vi "remote_fpga.vi"() -> ()   [LabVIEW 2018]
uses:
  packet_t.ctl
  packet_type_t.ctl
  spi_instructions.ctl
  seven_seg_digit.ctl
  grabber_register_addr.ctl
panel:
  out "unsigned byte array":u8[](array[numeric]) format="%x"
  out "Numeric":u8 format="%x"
  out "stop 3":bool
  in  "address":string="172.16.1.2"
  out "stop 2":bool
  in  "Colors [4]":cluster{u32, u32}[](array[cluster]) {"?" format="%x"}
  in  "stop":bool
  in  "Remote FPGA":enum32{"GPIO", "Page 2"}(tab)
  in  "Buttons":T1
  in  "SW7-0":bool[](array[boolean])=[FALSE, FALSE, FALSE, FALSE, FALSE, FALSE, FALSE, FALSE]
  in  "SW15-8":bool[](array[boolean])=[FALSE, FALSE, FALSE, FALSE, FALSE, FALSE, FALSE, FALSE]
  in  "Enable all":bool
  in  "Reset all":bool
  out "LED7-0":bool[](array[boolean])
  out "LED15-8":bool[](array[boolean])
  out "Digit":T2
  out "Digit 1":T2
  out "Digit 2":T2
  out "Digit 3":T2
  out "Digit 4":T2
  out "Digit 5":T2
  out "Digit 6":T2
  out "Digit 7":T2
  out "element":T3 {"instruction" items=["default"=0, "write"=173, "read"=237, "clear"=205]; "data" format="%x"; "address" format="%x"}
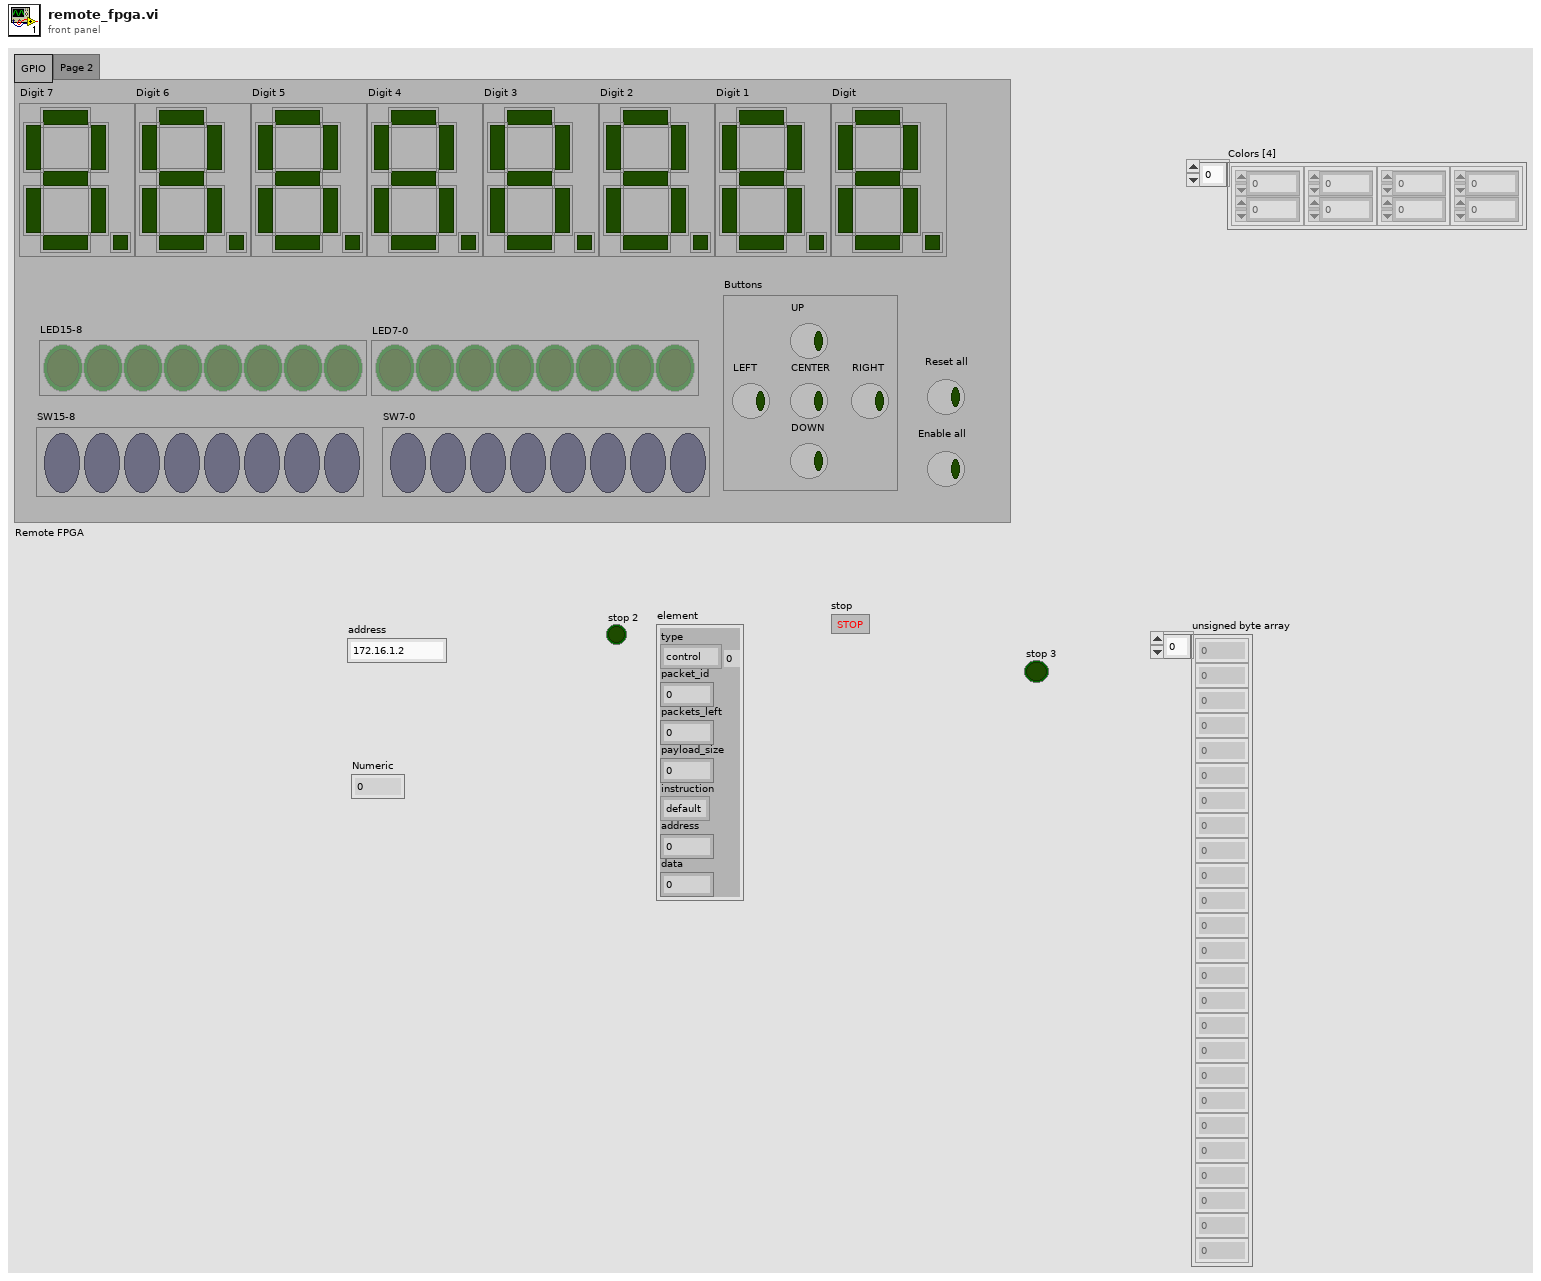
[diagram p1: front panel]
types:
  T1 = cluster{"CENTER":bool, "UP":bool, "LEFT":bool, "RIGHT":bool, "DOWN":bool}
  T2 = typedef "seven_seg_digit.ctl" = cluster{"DP":bool, "A":bool, "B":bool, "C":bool, "D":bool, "E":bool, "F":bool, "G":bool}
  T3 = typedef "packet_t.ctl" = cluster{"type":T4, "packet_id":u16, "packets_left":u16, "payload_size":u16, "instruction":T5, "address":u8, "data":u8}
  T4 = typedef "packet_type_t.ctl" = enum8{"control", "spi", "audio", "hdmi"}
  T5 = typedef "spi_instructions.ctl" = u8
  T6 = typedef "grabber_register_addr.ctl" = enum8{"rgb_data", "led_data_low", "led_data_high", "digit_0_data", "digit_1_data", "digit_2_data", "digit_3_data", "digit_4_data", "digit_5_data", "digit_6_data", "digit_7_data"}
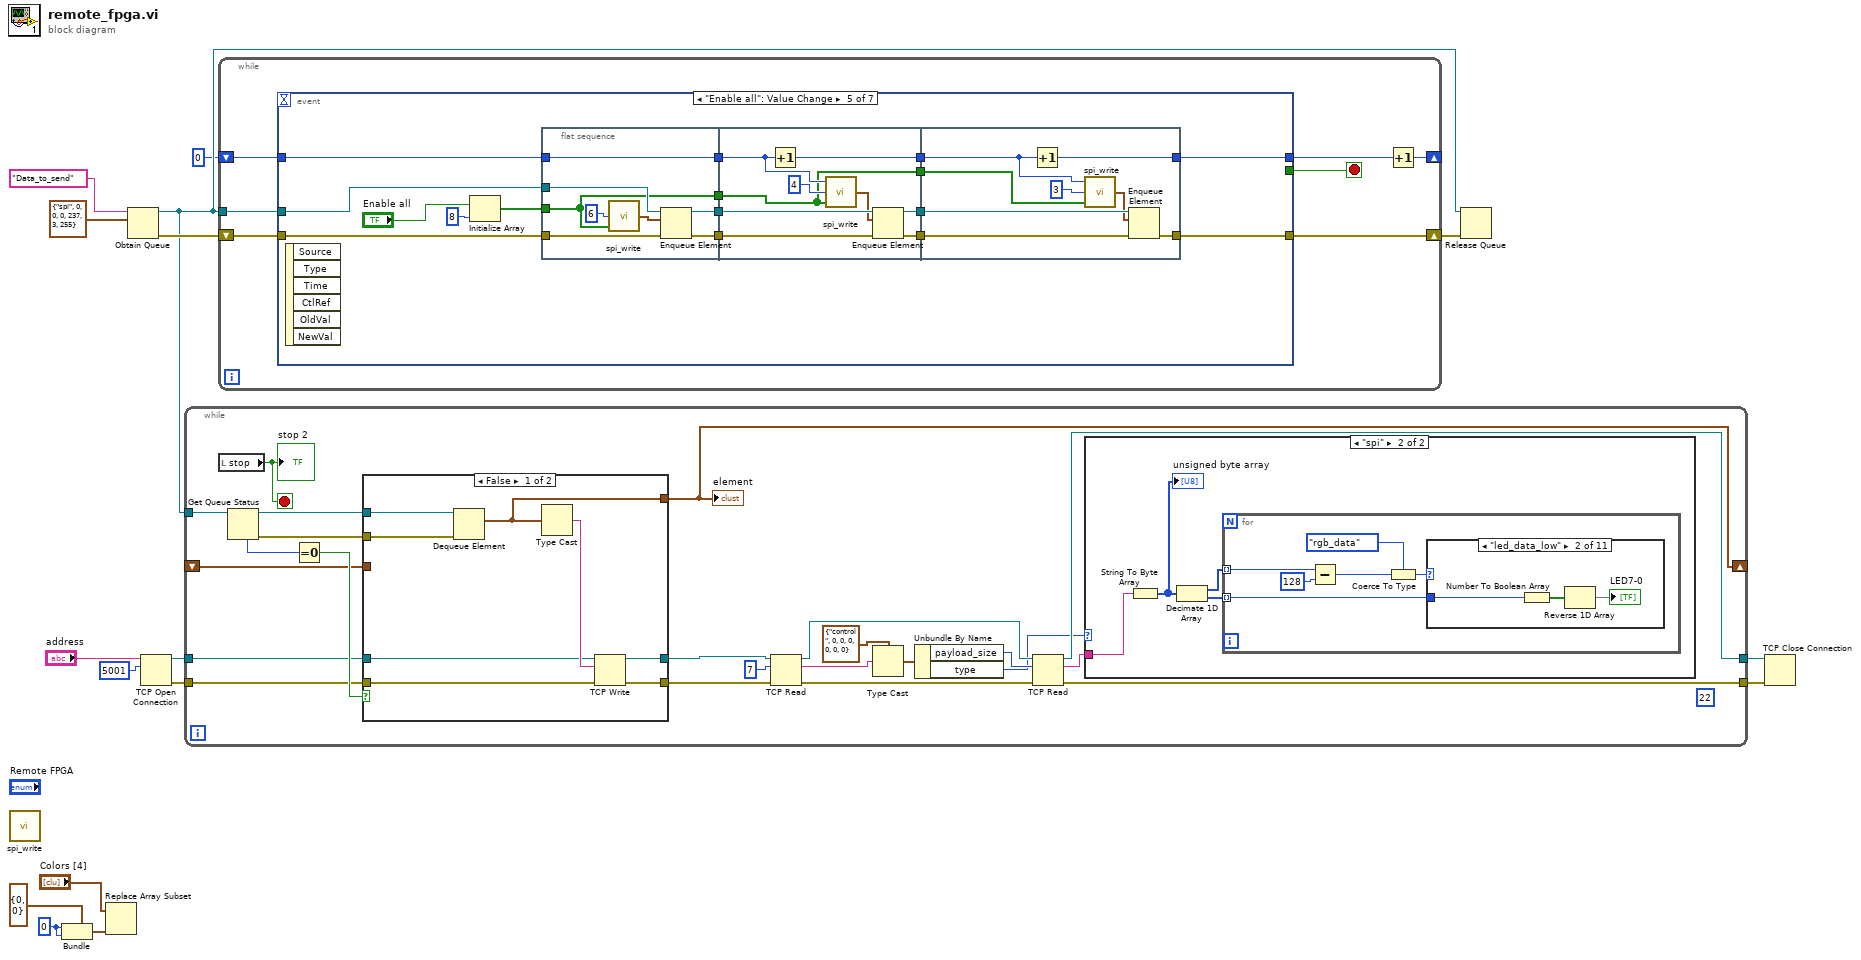
[diagram p0: block diagram]
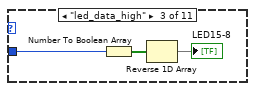
[diagram p4: hidden frame]
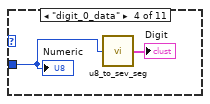
[diagram p5: hidden frame]
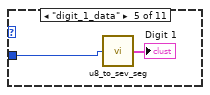
[diagram p6: hidden frame]
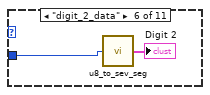
[diagram p7: hidden frame]
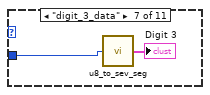
[diagram p8: hidden frame]
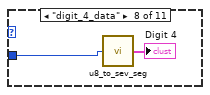
[diagram p9: hidden frame]
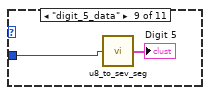
[diagram p10: hidden frame]
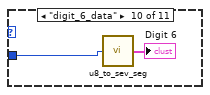
[diagram p11: hidden frame]
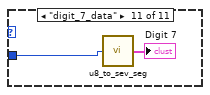
[diagram p12: hidden frame]
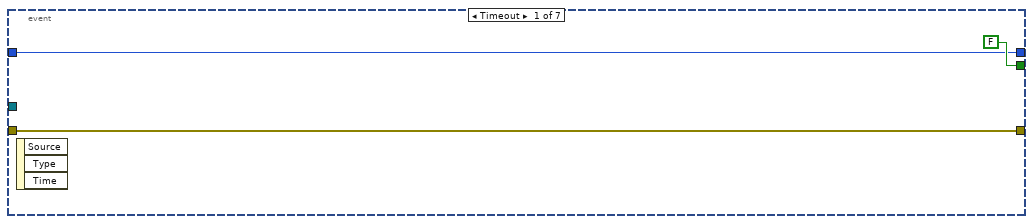
[diagram p14: hidden frame]
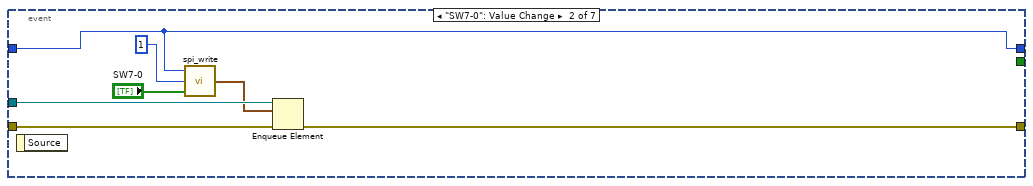
[diagram p15: hidden frame]
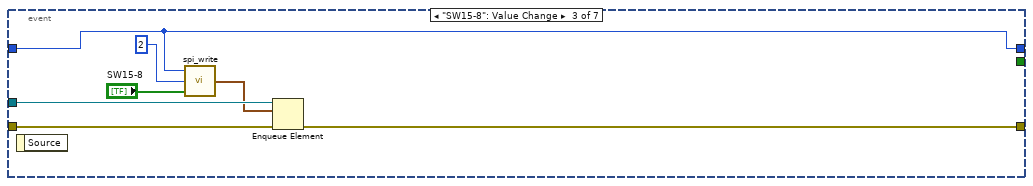
[diagram p16: hidden frame]
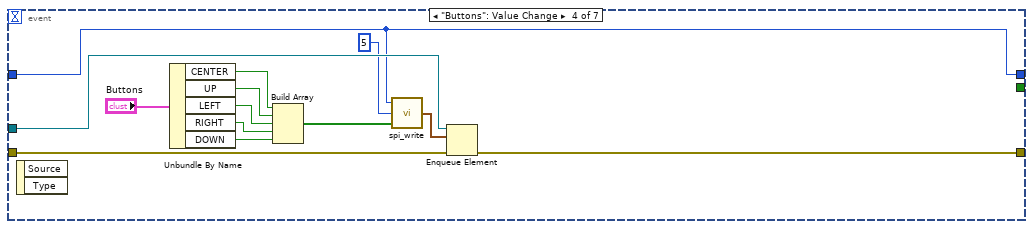
[diagram p17: hidden frame]
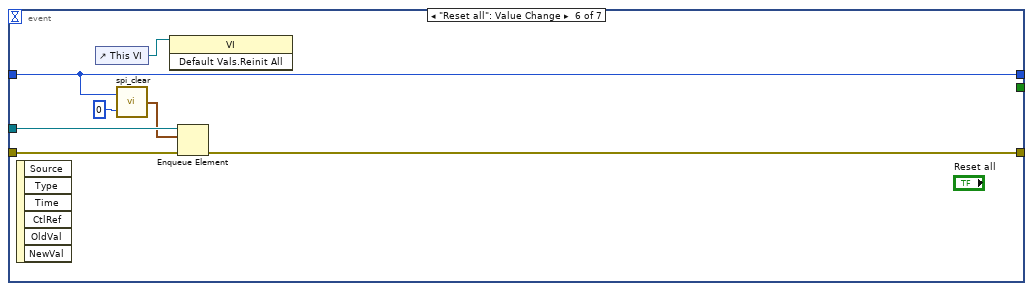
[diagram p18: hidden frame]
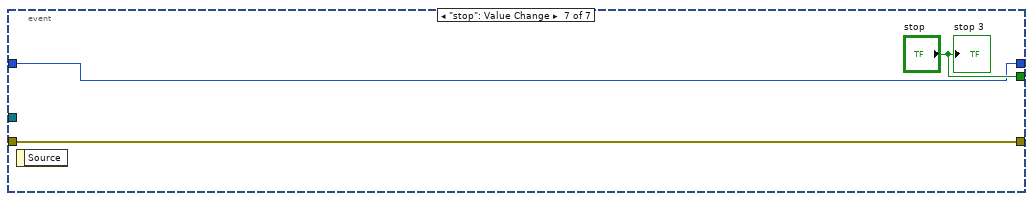
[diagram p19: hidden frame]
diagram:
  w13 = u32 0
  n1 = call "spi_write.vi"() -> ()  [unwired: 3 in, 1 out]
  n2 = Bundle(cluster=cluster{u32, u32} {0, 0}, w13, w13) -> (w16:cluster{u32, u32})
  n3 = Replace Array Subset(array="Colors [4]", new element=w16) -> ()  [unwired: 1 in, 1 out]
  n4 = Obtain Queue(name (unnamed)="Data_to_send", element data type=T3 {"type"=enum."spi", "packet_id"=0, "packets_left"=0, "payload_size"=0, "instruction"=237, "address"=3, "data"=255} ("packet_t")) -> (queue out=w8:refnum<queue>, error out=w10:errorcluster)  [unwired: 3 in, 1 out]
  n5 = TCP Open Connection(address="address", remote port or service name=u16 5001) -> (connection ID=w6:refnum<k5>, error out=w5:errorcluster)  [unwired: 3 in]
  n6 = while {
    tunnel: w8 -> [w38]
    tunnel: w6 -> [w33]
    tunnel: w5 -> [w32]
    shift-right: [w31] -> _
    shift-left: _ -> [w30]
    tunnel: [w19] -> w2
    tunnel: [w25] -> w1
    stop <- w39 stop-if-true
    (unwired) 22 ("bytes to read")
    n7 = local read "stop"() -> (w39:bool)
    "stop 2" <- w39
    n8 = Get Queue Status(queue=w38) -> (queue out=w36:refnum<queue>, error out=w35:errorcluster, # elements in queue=w37:i32)  [unwired: 2 in, 5 out]
    n9 = Equal To 0?(x=w37) -> (x = 0?=w34:bool)
    n10 = case shown="False" w34 {
      tunnel: w36 -> [w79 _]
      tunnel: w35 -> [w78 _]
      tunnel: w33 -> [w76 w82]
      tunnel: w32 -> [w75 w81]
      tunnel: [w74 w82] -> w26
      tunnel: [w73 w81] -> w24
      tunnel: [w72 w80] -> w31
      tunnel: w30 -> [_ w80]
      frame False {
        n11 = Dequeue Element(queue=w79, error in (no error)=w78) -> (element=w72:T3)  [unwired: 1 in, 3 out]
        n12 = Type Cast(x=w72) -> (*(type *) &x=w77:string)  [unwired: 1 in]
        n13 = TCP Write(connection ID=w76, data in=w77, error in (no error)=w75) -> (connection ID out=w74:refnum<k5>, error out=w73:errorcluster)  [unwired: 1 in, 1 out]
      }
      frame True {
      }
    }
    "element" <- w31
    n14 = TCP Read(connection ID=w26, bytes to read=7, error in (no error)=w24) -> (connection ID out=w28:refnum<k5>, data out=w21:string, error out=w29:errorcluster)  [unwired: 2 in]
    n15 = Type Cast(type=T3 {"type"=enum."control", "packet_id"=0, "packets_left"=0, "payload_size"=0, "instruction"=0, "address"=0, "data"=0} ("packet_t"), x=w21) -> (*(type *) &x=w22:T3)
    n16 = Unbundle By Name(w22) -> ("payload_size"=w18:u16, "type"=w17:T4)
    n17 = TCP Read(connection ID=w28, bytes to read=w18, error in (no error)=w29) -> (connection ID out=w19:refnum<k5>, data out=w20:string, error out=w25:errorcluster)  [unwired: 2 in]
    n18 = case shown="\"spi\"" w17 {
      tunnel: w20 -> [_ w43]
      frame "control", Default {
      }
      frame "spi" {
        n19 = String To Byte Array(string=w43) -> (unsigned byte array=w42:u8[])
        "unsigned byte array" <- w42
        n20 = Decimate 1D Array(w42) -> (w41:u8[], w40:u8[])
        n21 = for {
          tunnel: w41 -> [w45] mode=indexing
          tunnel: w40 -> [w49] mode=indexing
          n22 = Subtract(x=w45, y=u8 128 ("x")) -> (x-y=w46:u8)
          n23 = Coerce To Type(0:w46, 1:grabber_register_addr."rgb_data" ("Enum")) -> (2:w47:T6)
          n24 = case shown="\"led_data_low\"" w47 {
            tunnel: w49 -> [_ w52 w55 w57 w59 w61 w63 w65 w67 w69 w71]
            frame "rgb_data", Default {
            }
            frame "led_data_low" {
              n25 = Number To Boolean Array(number=w52) -> (Boolean array=w51:bool[])
              n26 = Reverse 1D Array(array=w51) -> (reversed array=→"LED7-0":bool[])
            }
            frame "led_data_high" {
              n27 = Number To Boolean Array(number=w55) -> (Boolean array=w54:bool[])
              n28 = Reverse 1D Array(array=w54) -> (reversed array=→"LED15-8":bool[])
            }
            frame "digit_0_data" {
              n29 = call "u8_to_sev_seg.vi"("Numeric"=w57) -> ("Digit"=→"Digit":T2)
              "Numeric" <- w57
            }
            frame "digit_1_data" {
              n30 = call "u8_to_sev_seg.vi"("Numeric"=w59) -> ("Digit"=→"Digit 1":T2)
            }
            frame "digit_2_data" {
              n31 = call "u8_to_sev_seg.vi"("Numeric"=w61) -> ("Digit"=→"Digit 2":T2)
            }
            frame "digit_3_data" {
              n32 = call "u8_to_sev_seg.vi"("Numeric"=w63) -> ("Digit"=→"Digit 3":T2)
            }
            frame "digit_4_data" {
              n33 = call "u8_to_sev_seg.vi"("Numeric"=w65) -> ("Digit"=→"Digit 4":T2)
            }
            frame "digit_5_data" {
              n34 = call "u8_to_sev_seg.vi"("Numeric"=w67) -> ("Digit"=→"Digit 5":T2)
            }
            frame "digit_6_data" {
              n35 = call "u8_to_sev_seg.vi"("Numeric"=w69) -> ("Digit"=→"Digit 6":T2)
            }
            frame "digit_7_data" {
              n36 = call "u8_to_sev_seg.vi"("Numeric"=w71) -> ("Digit"=→"Digit 7":T2)
            }
          }
        }
      }
    }
  }
  n37 = while {
    tunnel: w8 -> [w88]
    shift-right: [w86] -> w9
    shift-left: w10 -> [w87]
    shift-right: [w83] -> _
    shift-left: u16 0 -> [w85]
    stop <- w89 stop-if-true
    n38 = event shown="[4] \"Enable all\": Value Change" {
      selector: _ -> [_ _ _ _ _ _ _]
      dyn-events: _ -> [_ _ _ _ _ _ _]
      timeout: _ -> [_ _ _ _ _ _ _]
      tunnel: [FALSE ("stop") _ _ _ _ _ "stop"] -> w89
      tunnel: w88 -> [_ w99 w106 w119 w131 w167 _]
      tunnel: w87 -> [w90 w98 w105 w118 w135 w166 w168]
      tunnel: [w90 w97 w104 w117 w134 w165 w168] -> w86
      tunnel: [w91 w93 w101 w114 w125 w162 w169] -> w84
      tunnel: w85 -> [w91 w93 w101 w114 w127 w162 w169]
      event Timeout {
        n39 = event-data() -> ()  [unwired: 1 in, 3 out]
      }
      event "SW7-0": Value Change {
        n40 = event-data() -> ()  [unwired: 1 in, 1 out]
        n41 = call "spi_write.vi"("data"="SW7-0", "address"=u8 1 ("packets_left"), "packet_id"=w93) -> ("output cluster"=w96:T3)
        n42 = Enqueue Element(queue=w99, element=w96, error in (no error)=w98) -> (error out=w97:errorcluster)  [unwired: 1 in, 2 out]
      }
      event "SW15-8": Value Change {
        n43 = event-data() -> ()  [unwired: 1 in, 1 out]
        n44 = call "spi_write.vi"("data"="SW15-8", "address"=u8 2 ("packets_left"), "packet_id"=w101) -> ("output cluster"=w103:T3)
        n45 = Enqueue Element(queue=w106, element=w103, error in (no error)=w105) -> (error out=w104:errorcluster)  [unwired: 1 in, 2 out]
      }
      event "Buttons": Value Change {
        n46 = event-data() -> ()  [unwired: 1 in, 2 out]
        n47 = Unbundle By Name("Buttons") -> ("CENTER"=w112:bool, "UP"=w111:bool, "LEFT"=w110:bool, "RIGHT"=w109:bool, "DOWN"=w108:bool)
        n48 = Build Array(w112, w111, w110, w109, w108) -> (w107:bool[])
        n49 = call "spi_write.vi"("data"=w107, "address"=u8 5 ("packets_left"), "packet_id"=w114) -> ("output cluster"=w116:T3)
        n50 = Enqueue Element(queue=w119, element=w116, error in (no error)=w118) -> (error out=w117:errorcluster)  [unwired: 1 in, 2 out]
      }
      event "Enable all": Value Change {
        n51 = event-data() -> ()  [unwired: 1 in, 6 out]
        n52 = Initialize Array("Enable all", 8 ("dimension size")) -> (w122:bool[])
        n53 = flat-sequence {
          tunnel: w135 -> [w143]
          tunnel: [w142] -> w133
          tunnel: w131 -> [w140]
          tunnel: [w139] -> w129
          tunnel: [w137] -> w128
          tunnel: w127 -> [w137]
          tunnel: w122 -> [w136]
          tunnel: [w136] -> w121
          tunnel: w133 -> [w152]
          tunnel: [w151] -> w132
          tunnel: [w150] -> w130
          tunnel: w129 -> [w149]
          tunnel: w128 -> [w146]
          tunnel: [w147] -> w126
          tunnel: w121 -> [w144]
          tunnel: [w144] -> w120
          tunnel: [w159] -> w134
          tunnel: w132 -> [w160]
          tunnel: w130 -> [w158]
          tunnel: w126 -> [w155]
          tunnel: [w157] -> w125
          tunnel: w120 -> [w153]
          frame #0 {
            n54 = call "spi_write.vi"("data"=w136, "address"=u8 6 ("packets_left")) -> ("output cluster"=w138:T3)  [unwired: 1 in]
            n55 = Enqueue Element(queue=w140, element=w138, error in (no error)=w143) -> (queue out=w139:refnum<queue>, error out=w142:errorcluster)  [unwired: 1 in, 1 out]
          }
          frame #1 {
            n56 = Increment(x=w146) -> (x+1=w147:u16)
            n57 = call "spi_write.vi"("data"=w144, "address"=u8 4, "packet_id"=w146) -> ("output cluster"=w148:T3)
            n58 = Enqueue Element(queue=w149, element=w148, error in (no error)=w152) -> (queue out=w150:refnum<queue>, error out=w151:errorcluster)  [unwired: 1 in, 1 out]
          }
          frame #2 {
            n59 = Increment(x=w155) -> (x+1=w157:u16)
            n60 = call "spi_write.vi"("data"=w153, "address"=u8 3, "packet_id"=w155) -> ("output cluster"=w156:T3)
            n61 = Enqueue Element(queue=w158, element=w156, error in (no error)=w160) -> (error out=w159:errorcluster)  [unwired: 1 in, 2 out]
          }
        }
      }
      event "Reset all": Value Change {
        n62 = event-data() -> ()  [unwired: 1 in, 6 out]
        n63 = control-ref of="This VI"() -> (w161:refnum<vi>)
        n64 = call "spi_clear.vi"("address"=u8 0 ("packets_left"), "packet_id"=w162) -> ("output cluster"=w164:T3)
        n65 = invoke class="VI" method="Default Vals.Reinit All"(reference=w161) -> ()  [unwired: 2 in, 3 out]
        n66 = Enqueue Element(queue=w167, element=w164, error in (no error)=w166) -> (error out=w165:errorcluster)  [unwired: 1 in, 2 out]
      }
      event "stop": Value Change {
        n67 = event-data() -> ()  [unwired: 1 in, 1 out]
        "stop 3" <- "stop"
      }
    }
    n68 = Increment(x=w84) -> (x+1=w83:u16)
  }
  n69 = Release Queue(queue=w8, error in (no error)=w9) -> ()  [unwired: 1 in, 3 out]
  n70 = TCP Close Connection(connection ID=w2, error in (no error)=w1) -> ()  [unwired: 1 in, 2 out]
